vi "Git API.vi"(8 "error in (no error)":errorcluster, 11 "Git Updater Module in":refnum<class "Git Updater Module.lvclass">) -> (0 "error out":errorcluster, 2 "git-api":refnum<class "GIT-api.lvclass">, 3 "Git Updater Module out":refnum<class "Git Updater Module.lvclass">)   [LabVIEW 2020, in "VolatusGUI.lvlib" / "Git Updater Module.lvclass"]
uses:
  Git Updater Module.lvclass
  Git Updater Module.lvclass/Git Updater Module.ctl
  <vilib>/Hampel Software Engineering/Git API/Git API/GIT-api.lvclass
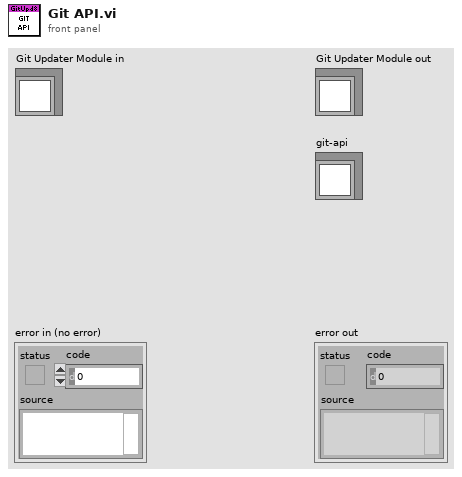
[diagram p1: front panel]
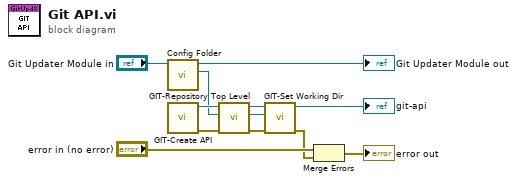
[diagram p0: block diagram]
diagram:
  n1 = call "Config Folder.vi"("Git Updater Module in"="Git Updater Module in") -> ("Config Folder"=w6:path, "Git Updater Module out"=→"Git Updater Module out":refnum<class "Git Updater Module.lvclass">)  [unwired: 8 in, 1 out]
  n2 = call <vilib>:"GIT-Create API.vi"() -> ("error out"=w10:errorcluster, "git-api out"=w11:refnum<class "GIT-api.lvclass">)  [unwired: 10 in]
  n3 = call <vilib>:"GIT-Repository Top Level.vi"("error in"=w10, "Current Path"=w6, "git-api in"=w11) -> ("error out"=w7:errorcluster, "Repo Top Level Path"=w8:path, "git-api out"=w9:refnum<class "GIT-api.lvclass">)  [unwired: 6 in]
  n4 = call <vilib>:"GIT-Set Working Dir.vi"("error in"=w7, "Working Directory"=w8, "git-api in"=w9) -> ("error out"=w2:errorcluster, "git-api out"=→"git-api":refnum<class "GIT-api.lvclass">)  [unwired: 7 in]
  n5 = Merge Errors("error in (no error)", w2) -> (→"error out":errorcluster)
